vi "Write JSON Response.vi"(8 "Error In":errorcluster, 10 "JSON Response":string, 11 "LabVIEW Web Service Request In":refnum<class "Web Request.lvclass">) -> (0 "Error Out":errorcluster, 3 "LabVIEW Web Service Request Out":refnum<class "Web Request.lvclass">)   [LabVIEW 2014, in "lvwd-components-start-utilities.lvlib"]
doc: "Takes a JSON string and writes the response on the Web Service Request object. \n\nIf an error message is passed in the VI returns an HTTP Status Code of Internal Error (500) and in the response body includes a JSON object with the error message and error cluster"
uses:
  lvwd-components-start-utilities.lvlib
  <vilib>/wsapi/Web Request.lvclass
  <vilib>/Utility/error.llb/DialogType.ctl
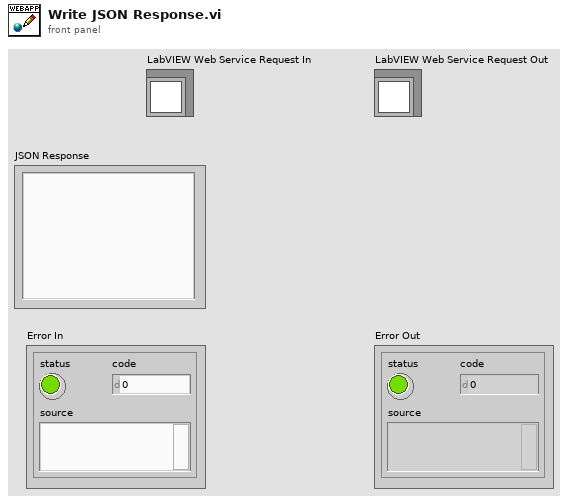
[diagram p1: front panel]
types:
  T1 = typedef "DialogType.ctl" = u16
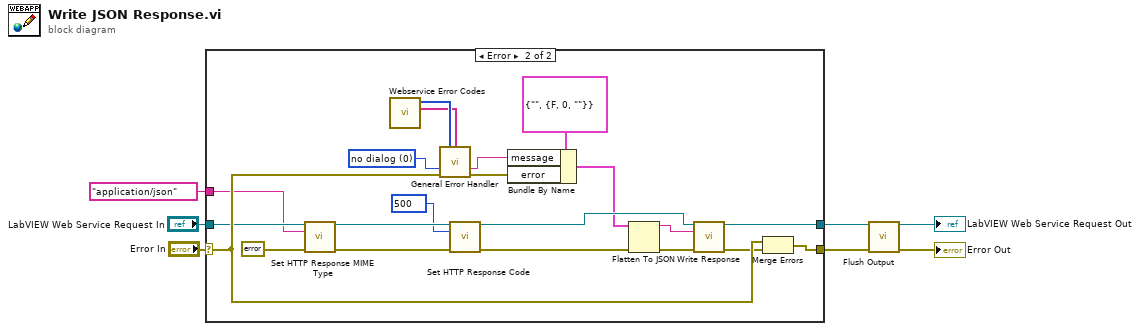
[diagram p0: block diagram]
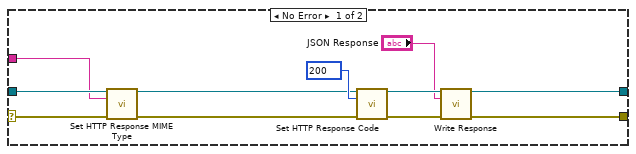
[diagram p2: hidden frame]
diagram:
  n1 = case shown="Error" "Error In" {
    selector: "Error In" -> [w9 w39]
    tunnel: [w14 w22] -> w7
    tunnel: [w13 w35] -> w6
    tunnel: "LabVIEW Web Service Request In" -> [w10 w29]
    tunnel: "application/json" ("MIME type (text/html)") -> [w8 w28]
    frame No Error {
      w15 = 200 items=["100"=100, "101"=101, "200"=200, "201"=201, "202"=202, "203"=203, "204"=204, "205"=205, "206"=206, "300"=300, "301"=301, "302"=302, "303"=303, "304"=304, "305"=305, "306"=306, "307"=307, "400"=400, "401"=401, "402"=402, "403"=403, "404"=404, "405"=405, "406"=406, "407"=407, "408"=408, "409"=409, "410"=410, "411"=411, "412"=412, "413"=413, "414"=414, "415"=415, "416"=416, "417"=417, "500"=500, "501"=501, "502"=502, "503"=503, "504"=504, "505"=505] ("response code")
      n2 = call <vilib>:"Set HTTP Response MIME Type.vi"("LabVIEW Web Service Request"=w10, "MIME type (text/html)"=w8, "error in (no error)"=w9) -> ("LabVIEW Web Service Request out"=w11:refnum<class "Web Request.lvclass">, "error out"=w12:errorcluster)  [unwired: 11 in]
      n3 = call <vilib>:"Set HTTP Response Code.vi"("LabVIEW Web Service Request"=w11, "response code (200)"=w15, "error in (no error)"=w12) -> ("LabVIEW Web Service Request out"=w18:refnum<class "Web Request.lvclass">, "error out"=w16:errorcluster)  [unwired: 11 in]
      n4 = call <vilib>:"Write Response.vi"("LabVIEW Web Service Request"=w18, "response string"="JSON Response", "error in (no error)"=w16) -> ("LabVIEW Web Service Request out"=w13:refnum<class "Web Request.lvclass">, "error out"=w14:errorcluster)  [unwired: 11 in]
    }
    frame Error {
      w27 = T1 0 items=["no dialog", "OK message", "continue or stop message", "OK message + warnings", "continue/stop + warnings"] ("type of dialog (OK msg:1)")
      w36 = 500 items=["100"=100, "101"=101, "200"=200, "201"=201, "202"=202, "203"=203, "204"=204, "205"=205, "206"=206, "300"=300, "301"=301, "302"=302, "303"=303, "304"=304, "305"=305, "306"=306, "307"=307, "400"=400, "401"=401, "402"=402, "403"=403, "404"=404, "405"=405, "406"=406, "407"=407, "408"=408, "409"=409, "410"=410, "411"=411, "412"=412, "413"=413, "414"=414, "415"=415, "416"=416, "417"=417, "500"=500, "501"=501, "502"=502, "503"=503, "504"=504, "505"=505] ("response code")
      n5 = call <vilib>:"Set HTTP Response MIME Type.vi"("LabVIEW Web Service Request"=w29, "MIME type (text/html)"=w28, "error in (no error)"=errorcluster {"status"=FALSE, "code"=0, "source"=""}) -> ("LabVIEW Web Service Request out"=w38:refnum<class "Web Request.lvclass">, "error out"=w32:errorcluster)  [unwired: 11 in]
      n6 = call "Webservice Error Codes.vi"() -> ("webservice error descriptions"=w19:string[], "webservice error codes"=w20:i32[])  [unwired: 10 in]
      n7 = call <vilib>:"General Error Handler.vi"("[user-defined codes]"=w20, "[user-defined descriptions]"=w19, "type of dialog (OK msg:1)"=w27, "error in (no error)"=w39) -> ("message"=w25:string, "error out"=w24:errorcluster)  [unwired: 7 in, 3 out]
      n8 = call <vilib>:"Set HTTP Response Code.vi"("LabVIEW Web Service Request"=w38, "response code (200)"=w36, "error in (no error)"=w32) -> ("LabVIEW Web Service Request out"=w37:refnum<class "Web Request.lvclass">, "error out"=w30:errorcluster)  [unwired: 11 in]
      n9 = Bundle By Name(cluster=cluster{"message":string, "error":errorcluster} {"message"="", "error"={"status"=FALSE, "code"=0, "source"=""}}, "message"=w25, "error"=w24) -> (w23:cluster{"message":string, "error":errorcluster})
      n10 = Flatten To JSON(anything=w23, error in (no error)=w30) -> (JSON string=w33:string, 11:w34:errorcluster)  [unwired: 1 in]
      n11 = call <vilib>:"Write Response.vi"("LabVIEW Web Service Request"=w37, "response string"=w33, "error in (no error)"=w34) -> ("LabVIEW Web Service Request out"=w35:refnum<class "Web Request.lvclass">, "error out"=w21:errorcluster)  [unwired: 11 in]
      n12 = Merge Errors(w39, w21) -> (w22:errorcluster)
    }
  }
  n13 = call <vilib>:"Flush Output.vi"("LabVIEW Web Service Request"=w6, "error in (no error)"=w7) -> ("LabVIEW Web Service Request out"=→"LabVIEW Web Service Request Out":refnum<class "Web Request.lvclass">, "error out"=→"Error Out":errorcluster)  [unwired: 12 in]
